vi "Robot Global Data.vi"() -> ()   [LabVIEW 2018]
doc: "This global VI can contain as many global variables as you need. Place a control on the panel, give it a good name. To read or write to it from a VI, drag the icon to the diagram of that VI. You can also drag from the project. Click on the node to change which global you access. You shouldn't have multiple locations writing to a global or it will cause a race-condition."
uses:
  <vilib>/Rock Robotics/WPI/Camera/WPI_CameraImageSize.ctl
  <vilib>/Rock Robotics/WPI/DriverStation/WPI_DriverStationRobotMode2.ctl
panel:
  out "Left Encoder Count":dbl
  out "Right Encoder Count":dbl
  in  "Vision Toggle":bool
  in  "Tomahawk":bool
  in  "Level Up":bool
  in  "Cargo OUT":bool
  in  "Cargo IN":bool
  in  "Lift Auto/Man":bool
  in  "Top Position":bool
  in  "Middle Position":bool
  in  "Bottom Position":bool
  out "Direction":dbl
  out "Acceleration":dbl
  out "Ball Collector":dbl
  in  "Cargo Arm UP/DOWN":bool
  out "Climb":dbl
  in  "Intake Slide":bool
  in  "Hatch In/Out":bool
  in  "Robot Direction":bool
  out "Right Y-axis":dbl
  out "Left Y-Axis":dbl
  in  "Robot Mode":T1
  in  "image size":T2=enum."320x240"
  in  "Enable Vision":bool
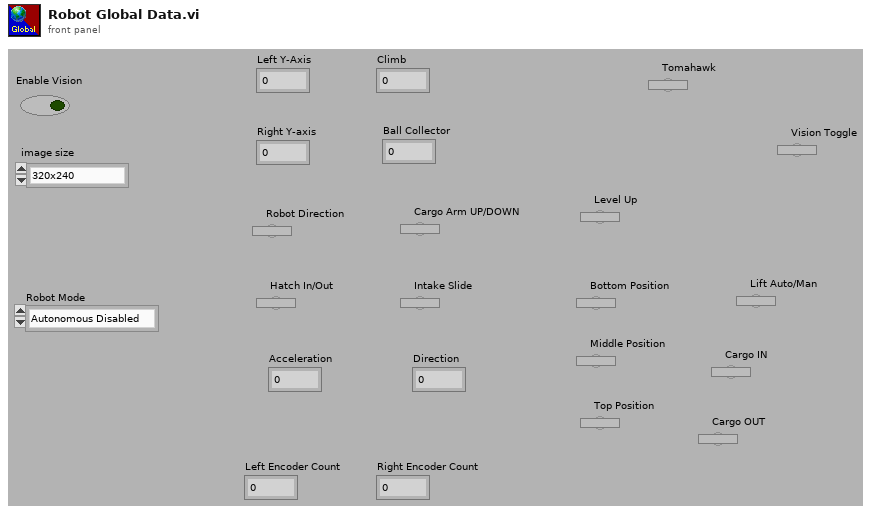
[diagram p1: front panel]
types:
  T1 = typedef "WPI_DriverStationRobotMode2.ctl" = enum16{"Autonomous Disabled", "Autonomous Enabled", "Teleop Disabled", "Teleop Enabled", "Disconnected", "Finish", "Test Disabled", "Test Enabled", "Emergency Stopped"}
  T2 = typedef "WPI_CameraImageSize.ctl" = enum16{"640x480", "320x240", "160x120", "Custom"}
diagram:
